vi "SPL meter RMS.vi"() -> ()   [LabVIEW 2018]
panel:
  in  "Start/Stop":bool
  in  "Filename":path=path "tdms"
  out "Sound Level":bool
  in  "Fast/Slow":bool caption="Blank Button"
  in  "Off":bool
  in  "Open":bool
  out "Meter":dbl(knob) scale=30.0..90.0
  out "Waveform Chart":waveform(dbl)(graph)
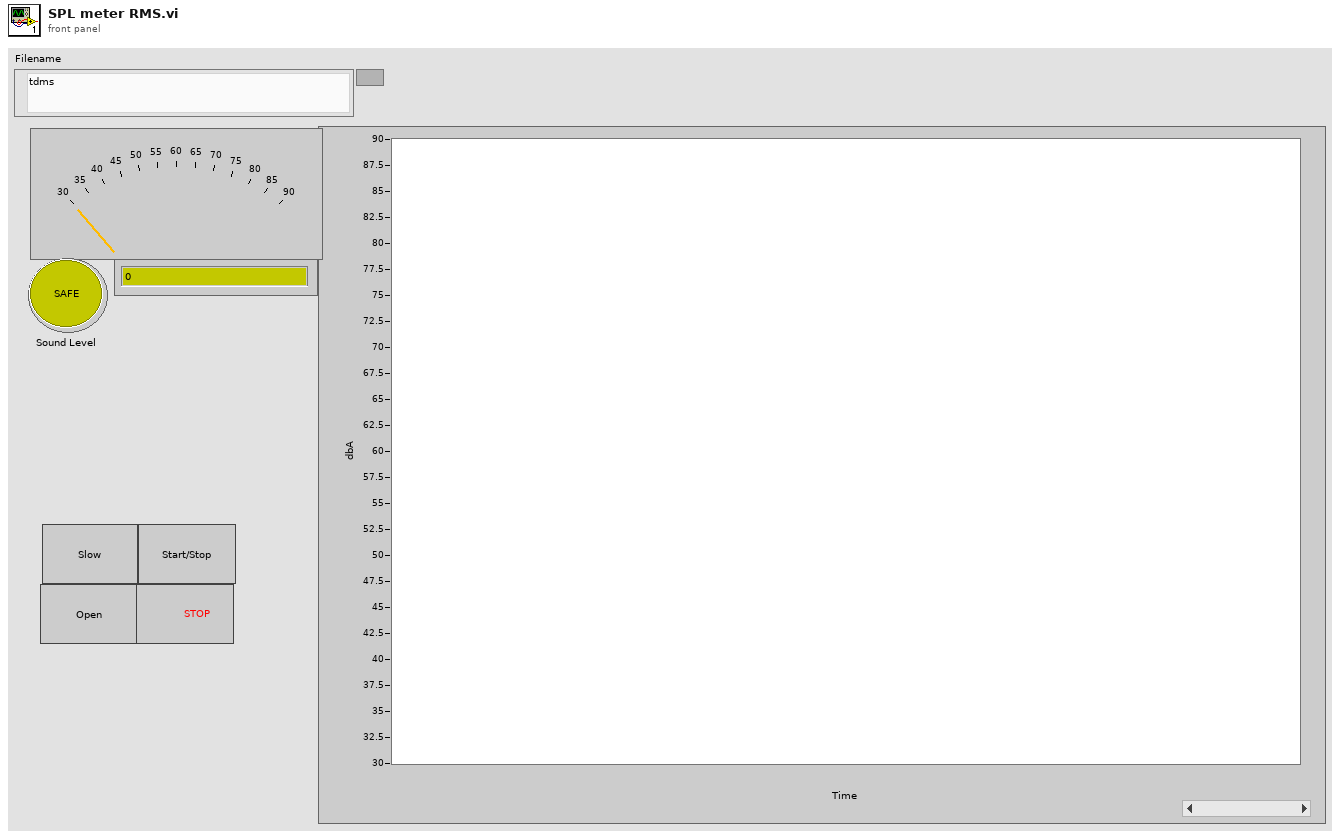
[diagram p1: front panel]
types:
  T1 = enum8{"Enabled", "Disabled", "Disabled and Grayed Out"}
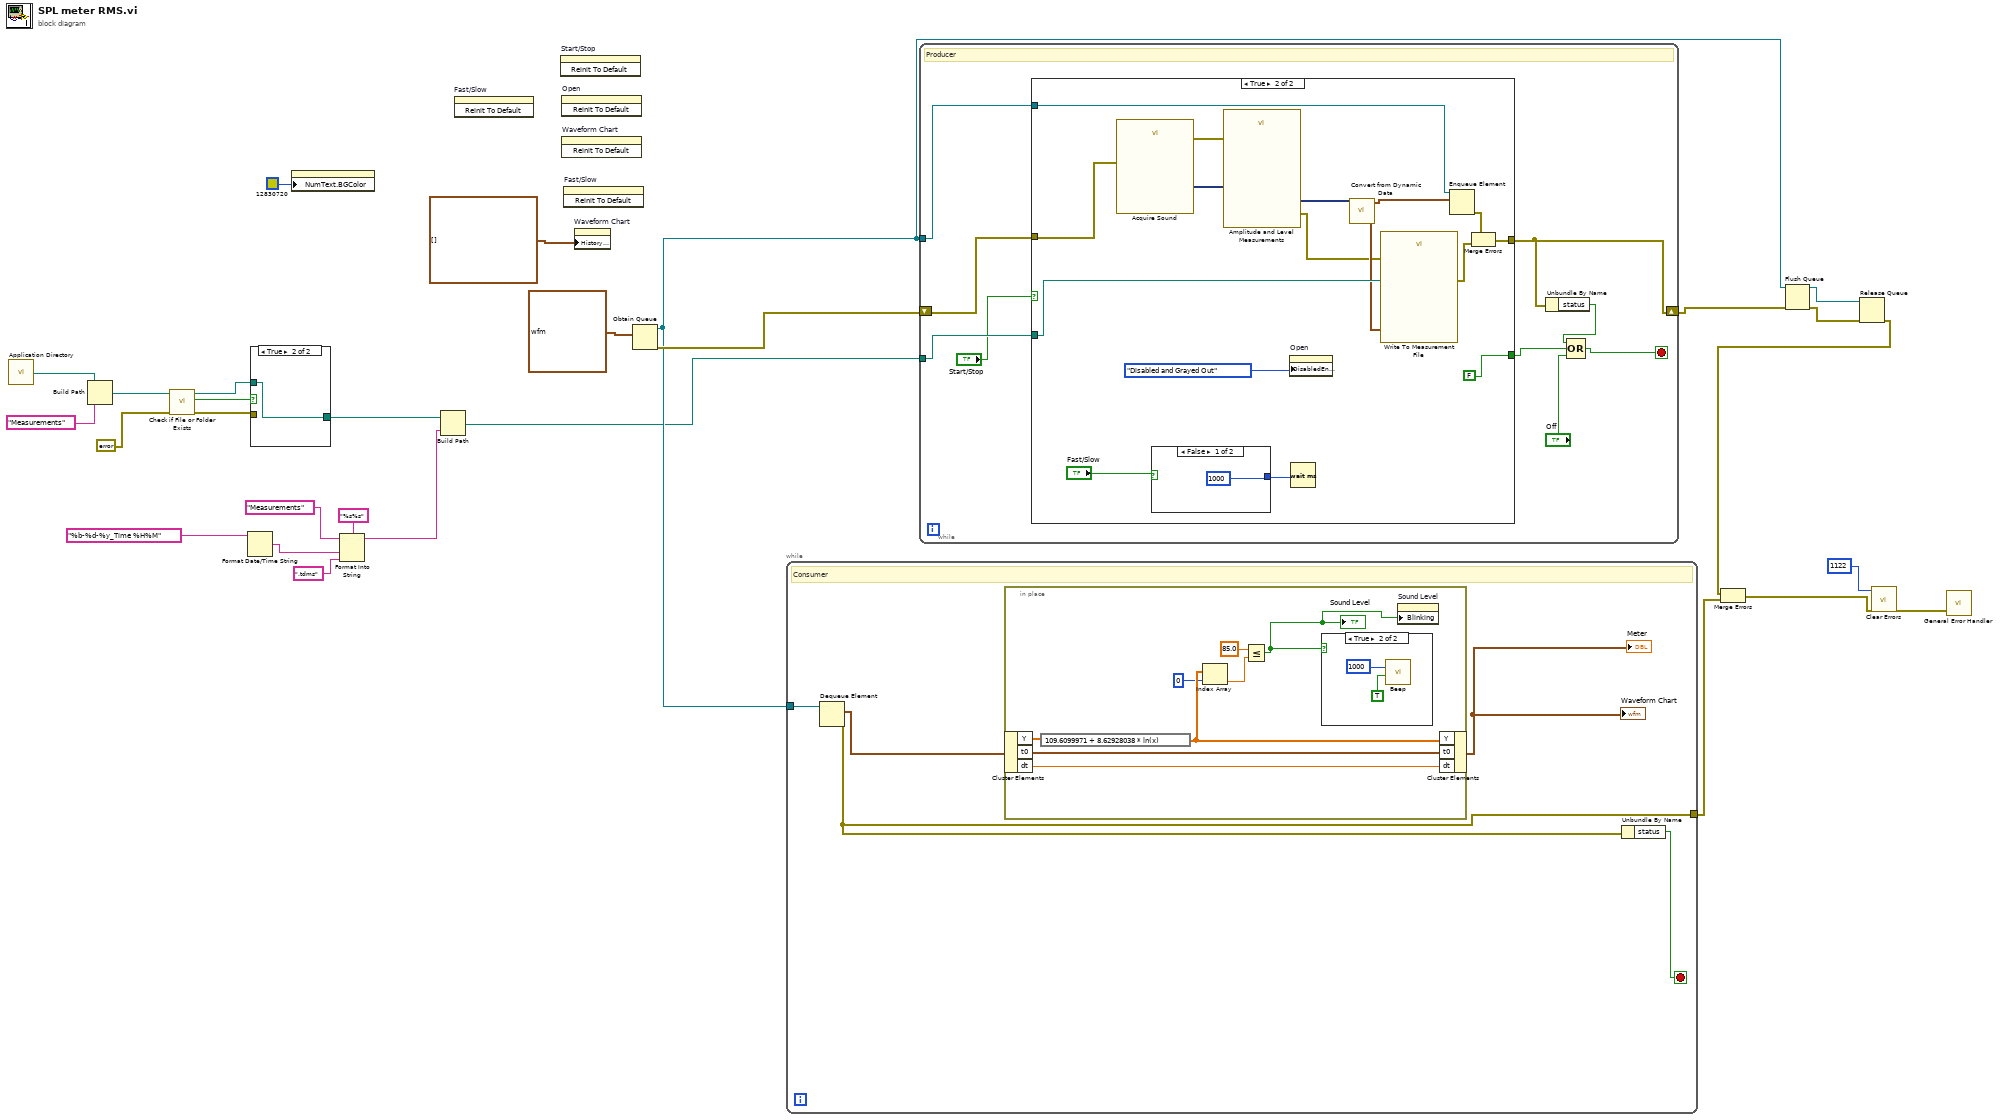
[diagram p0: block diagram]
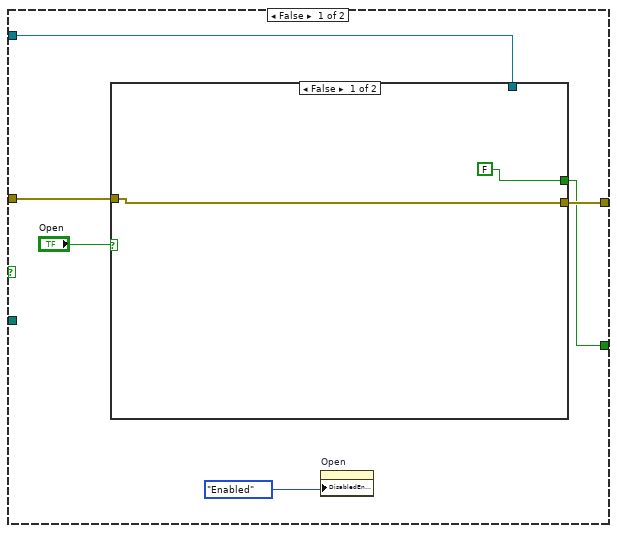
[diagram p3: hidden frame]
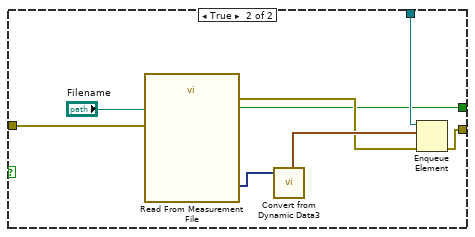
[diagram p4: hidden frame]
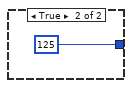
[diagram p5: hidden frame]
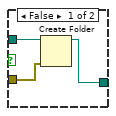
[diagram p6: hidden frame]
diagram:
  n1 = call <vilib>:"Application Directory.vi"() -> ("Application Directory"=w28:path)
  n2 = Build Path(base path=w28, name or relative path="Measurements") -> (appended path=w20:path)
  n3 = call <vilib>:"Check if File or Folder Exists.vi"("error in (no error)"=errorcluster {"status"=FALSE, "code"=0, "source"=""} ("error in"), "path"=w20) -> ("error out"=w15:errorcluster, "file or folder exists?"=w18:bool, "dup path"=w16:path)  [unwired: 7 in]
  n4 = Format Date/Time String(time format string (%c)="%b-%d-%y_Time %H%M") -> (date/time string=w23:string)  [unwired: 2 in]
  n5 = case shown="True" w18 {
    tunnel: [w31 w32] -> w17
    tunnel: w16 -> [w30 w32]
    tunnel: w15 -> [w29 _]
    frame False {
      n6 = Create Folder(path (use dialog)=w30, error in=w29) -> (created path=w31:path)  [unwired: 1 in, 2 out]
    }
    frame True {
    }
  }
  n7 = property class="DigNum (strict)"("NumText.BGColor"=u32 12830720) -> ()  [unwired: 2 in, 2 out]
  n8 = Format Into String(format string="%s%s", initial string="Measurements", w23, ".tdms" ("input 2")) -> (resulting string=w21:string)  [unwired: 1 in, 1 out]
  n9 = Build Path(base path=w17, name or relative path=w21) -> (appended path=w3:path)
  n10 = invoke on="Fast/Slow" class="Bool (strict)" method="Reinit To Default"() -> ()  [unwired: 3 in, 3 out]
  n11 = invoke on="Start/Stop" class="Bool (strict)" method="Reinit To Default"() -> ()  [unwired: 3 in, 3 out]
  n12 = invoke on="Open" class="Bool (strict)" method="Reinit To Default"() -> ()  [unwired: 3 in, 3 out]
  n13 = invoke on="Waveform Chart" class="WFChart (strict)" method="Reinit To Default"() -> ()  [unwired: 3 in, 3 out]
  n14 = invoke on="Fast/Slow" class="Bool (strict)" method="Reinit To Default"() -> ()  [unwired: 3 in, 3 out]
  n15 = property on="Waveform Chart" class="WFChart (strict)"("History Data"=waveform(dbl)[] []) -> ()  [unwired: 2 in, 2 out]
  n16 = Obtain Queue(element data type=waveform(dbl) {"t0"=timestamp(0 s since 1904-01-01), "dt"=1.0, "Y"=[]} ("waveform")) -> (queue out=w6:refnum<queue>, error out=w13:errorcluster)  [unwired: 4 in, 1 out]
  n17 = while {
    tunnel: [w35] -> w12
    tunnel: w6 -> [w37]
    stop <- w34 stop-if-true
    # "Consumer"
    n18 = Dequeue Element(queue=w37) -> (element=w36:waveform(dbl), error out=w35:errorcluster)  [unwired: 2 in, 2 out]
    n19 = in-place {
      n20 = in-place-cluster #1(w36) -> ("Y"=w43:dbl[], "t0"=w45:timestamp, "dt"=w44:dbl)
      n21 = expression code="109.6099971 + 8.62928038 * ln(x)"(w43) -> (w42:dbl[])
      n22 = Index Array(array=w42, index=0) -> (element=w40:dbl)
      n23 = Less Or Equal?(x=85.0, y=w40) -> (x <= y?=w38:bool)
      "Sound Level" <- w38
      n24 = case shown="True" w38 {
        frame False {
        }
        frame True {
          n25 = call <vilib>:"Beep.vi"("use system alert? (T)"=TRUE, "duration (msec)"=u32 1000) -> ()  [unwired: 10 in]
        }
      }
      n26 = property on="Sound Level" class="Bool (strict)"("Blinking"=w38) -> ()  [unwired: 2 in, 2 out]
      n27 = in-place-cluster #1("Y"=w42, "t0"=w45, "dt"=w44) -> (→"Waveform Chart" →"Meter":waveform(dbl))
    }
    n28 = Unbundle By Name(w35) -> ("status"=w34:bool)
  }
  n29 = while "Producer Loop" {
    shift-right: [w52] -> w5
    shift-left: w13 -> [w56]
    tunnel: w6 -> [w55]
    tunnel: w3 -> [w54]
    stop <- w48 stop-if-true
    # "Producer"
    n30 = case shown="True" "Start/Stop" {
      tunnel: w56 -> [w61 w87]
      tunnel: w55 -> [w60 w86]
      tunnel: w54 -> [_ w85]
      tunnel: [w59 w77] -> w52
      tunnel: [w57 FALSE] -> w50
      frame False {
        n31 = case shown="False" "Open" {
          tunnel: w61 -> [w64 w68]
          tunnel: w60 -> [_ w67]
          tunnel: [w64 w66] -> w59
          tunnel: [FALSE w65] -> w57
          frame False {
          }
          frame True {
            n32 = call "Read From Measurement File"("error in (no error)"=w68, "Filename"="Filename") -> ("error out"=w71:errorcluster, "Signals"=w69:dynamicdata, "EOF?"=w65:bool)  [unwired: 4 in, 3 out]
            n33 = call "Convert from Dynamic Data3"("Dynamic Data Type"=w69) -> ("Waveform"=w72:waveform(dbl))  [unwired: 3 in]
            n34 = Enqueue Element(queue=w67, element=w72, error in (no error)=w71) -> (error out=w66:errorcluster)  [unwired: 1 in, 2 out]
          }
        }
        n35 = property on="Open" class="Bool (strict)"("DisabledEnum"=T1."Enabled" ("Disabled")) -> ()  [unwired: 2 in, 2 out]
      }
      frame True {
        n36 = call "Acquire Sound"("error in (no error)"=w87) -> ("Data"=w83:dynamicdata, "error out"=w84:errorcluster)  [unwired: 17 in]
        n37 = case shown="False" "Fast/Slow" {
          tunnel: [1000 u32 125 ("milliseconds to wait")] -> w75
          frame False {
          }
          frame True {
          }
        }
        n38 = call "Amplitude and Level Measurements"("Signals"=w83, "error in (no error)"=w84) -> ("RMS"=w82:dynamicdata, "error out"=w80:errorcluster)  [unwired: 12 in]
        n39 = property on="Open" class="Bool (strict)"("DisabledEnum"=T1."Disabled and Grayed Out" ("Disabled")) -> ()  [unwired: 2 in, 2 out]
        n40 = Wait (ms)(milliseconds to wait=w75) -> ()  [unwired: 1 out]
        n41 = call "Convert from Dynamic Data"("Dynamic Data Type"=w82) -> ("Waveform"=w81:waveform(dbl))  [unwired: 3 in]
        n42 = call "Write To Measurement File"("Signals"=w81, "error in (no error)"=w80, "Filename"=w85) -> ("error out"=w78:errorcluster)  [unwired: 14 in, 2 out]
        n43 = Enqueue Element(queue=w86, element=w81) -> (error out=w79:errorcluster)  [unwired: 2 in, 2 out]
        n44 = Merge Errors(w79, w78) -> (w77:errorcluster)
      }
    }
    n45 = Unbundle By Name(w52) -> ("status"=w51:bool)
    n46 = Compound Arithmetic op=OR(w51, w50, "Off") -> (w48:bool)
  }
  n47 = Flush Queue(queue=w6, error in (no error)=w5) -> (queue out=w7:refnum<queue>, error out=w4:errorcluster)  [unwired: 1 out]
  n48 = Release Queue(queue=w7, error in (no error)=w4) -> (error out=w10:errorcluster)  [unwired: 1 in, 2 out]
  n49 = Merge Errors(w10, w12) -> (w9:errorcluster)
  n50 = call <vilib>:"Clear Errors.vi"("error in (no error)"=w9, "specific error code to clear (0: all)"=1122) -> ("error out"=w11:errorcluster)  [unwired: 4 in, 1 out]
  n51 = call <vilib>:"General Error Handler.vi"("error in (no error)"=w11) -> ()  [unwired: 10 in, 5 out]
